vi "status_to_states.vi"(7 "actual value":u32) -> (8 "motion_state":T1=enum."CONST", 10 "other_states":T1[](array[typedef]))   [LabVIEW 2012]
doc: "This utility VI takes as input the value read as a result of an issued \"MST\" command and parses it accordingly. There are two types of states the device can be in. One is a motion based state, where the device can be in only one of these states:\n\n(1) Idle (IDLE)\n(2) Running at constant speed (CONST)\n(3) Accelerating (ACCEL)\n(4) Decelerating (DECEL)\n\nThe other is non-motion based, where multiple states can exist at one time (in addition to the single motion state above)\n\nNOTE: if any of the following states exist in the \"other_states\" array output, then they are considered logically TRUE\n\n(1) Home input switch status (HOME_SWITCH)\n(2) Minus limit input switch status (-LIMIT_SWITCH)\n(3) Plus limit input switch status (+LIMIT_SWITCH)\n(4) Minus limit error (-LIMIT_ERR)\n(5) Plus limit error (+LIMIT_ERR)\n(6) Communication timeout counter alarm (COMM_ERR)\n\nProduced By:\n\nChristopher Lemieux\nKod Integrations, LLC\n4835 Marianne Drive\nMount Airy, MD 21771\nhttp://www.kodintegrations.com\nemail: clemieux@kodintegrations.com\nphone: (240) 687-1288"
uses:
  controls/status_states.ctl
panel:
  out "other state":bool[](array[boolean])
  out "motion state":bool[](array[boolean])
  out "actual bits":bool[](array[boolean])
  # "constant"
  # "constant"
  # "accel"
  # "accel"
  # "decel"
  # "decel"
  # "home input switch"
  # "minus limit switch"
  # "home input switch"
  # "plus limit switch"
  # "minus limit switch"
  # "minus limit error"
  # "plus limit switch"
  # "plus limit error"
  # "minus limit error"
  # "n/a"
  # "plus limit error"
  # "n/a"
  # "timeout counter alarm"
  # "timeout counter alarm"
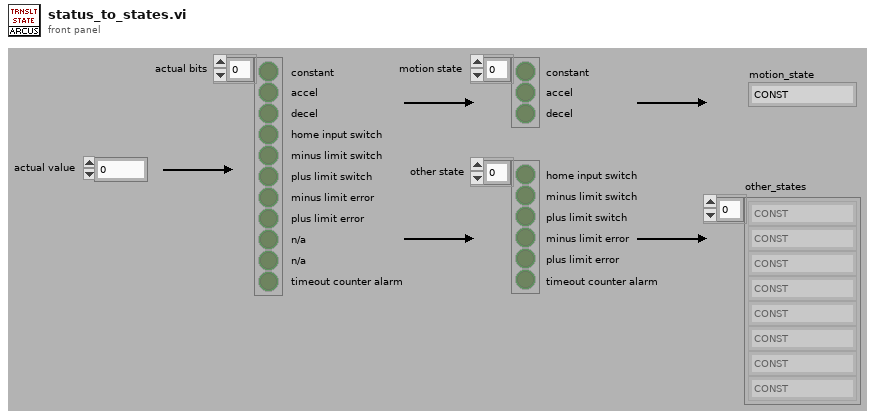
[diagram p1: front panel]
types:
  T1 = typedef "status_states.ctl" = enum16{"IDLE", "CONST", "ACCEL", "DECEL", "HOME_SWITCH", "-LIMIT_SWITCH", "+LIMIT_SWITCH", "-LIMIT_ERR", "+LIMIT_ERR", "COMM_ERR"}
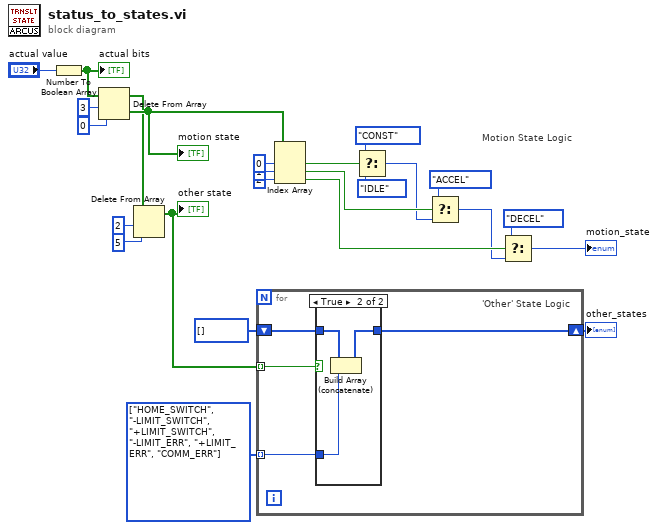
[diagram p0: block diagram]
diagram:
  w6 = T1[] [enum."HOME_SWITCH", enum."-LIMIT_SWITCH", enum."+LIMIT_SWITCH", enum."-LIMIT_ERR", enum."+LIMIT_ERR", enum."COMM_ERR"] items=["IDLE", "CONST", "ACCEL", "DECEL", "HOME_SWITCH", "-LIMIT_SWITCH", "+LIMIT_SWITCH", "-LIMIT_ERR", "+LIMIT_ERR", "COMM_ERR"]
  w7 = T1[] [] items=["IDLE", "CONST", "ACCEL", "DECEL", "HOME_SWITCH", "-LIMIT_SWITCH", "+LIMIT_SWITCH", "-LIMIT_ERR", "+LIMIT_ERR", "COMM_ERR"]
  # "Motion State Logic"
  n1 = Number To Boolean Array(number="actual value") -> (Boolean array=w24:bool[])
  "actual bits" <- w24
  n2 = Delete From Array(array=w24, length=3, index=0) -> (deleted portion=w8:bool[], array with subset deleted=w4:bool[])
  "motion state" <- w8
  n3 = Delete From Array(array=w4, length=2, index=5 ("length")) -> (array with subset deleted=w1:bool[])  [unwired: 1 out]
  "other state" <- w1
  n4 = for {
    tunnel: w1 -> [w29] mode=indexing
    shift-right: [w26] -> w5
    shift-left: w7 -> [w28]
    tunnel: w6 -> [w27] mode=indexing
    # "'Other' State Logic"
    n5 = case shown="True" w29 {
      tunnel: w28 -> [w30 w33]
      tunnel: w27 -> [_ w32]
      tunnel: [w30 w31] -> w26
      frame False {
      }
      frame True {
        n6 = Build Array (concatenate)(w33, w32) -> (w31:T1[])
      }
    }
  }
  "other_states" <- w5
  n7 = Index Array(array=w8, index #1=0 ("index"), index #2=1 ("index"), index #3=2 ("index")) -> (element #1=w17:bool, element #2=w15:bool, element #3=w11:bool)
  n8 = Select(t=status_states."CONST" ("motion_state"), s=w17, f=status_states."IDLE" ("motion_state")) -> (s? t:f=w14:T1)
  n9 = Select(t=status_states."ACCEL" ("motion_state"), s=w15, f=w14) -> (s? t:f=w10:T1)
  n10 = Select(t=status_states."DECEL" ("motion_state"), s=w11, f=w10) -> (s? t:f=→"motion_state":T1)
